vi "FPGA_Generate_PWM.vi"(10 "high-time (ticks)":i32, 11 "period(ticks)":i32) -> (3 "PWM out":bool)   [LabVIEW 2025]
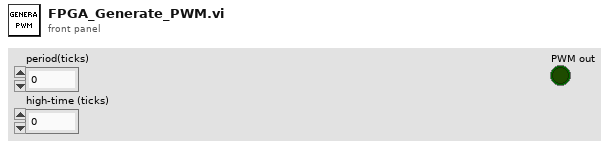
[diagram p1: front panel]
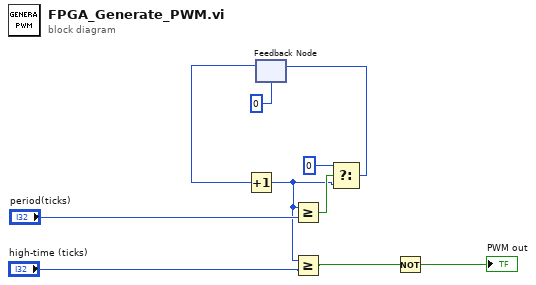
[diagram p0: block diagram]
diagram:
  n1 = feedback #1(0) -> (w9:i32)
  n2 = Increment(x=w9) -> (x+1=w4:i32)
  n3 = Greater Or Equal?(x=w4, y="period(ticks)") -> (x >= y?=w7:bool)
  n4 = Greater Or Equal?(x=w4, y="high-time (ticks)") -> (x >= y?=w2:bool)
  n5 = Select(t=0, s=w7, f=w4) -> (s? t:f=w5:i32)
  n6 = feedback-in #1(w5) -> ()
  n7 = Not(x=w2) -> (.not. x?=→"PWM out":bool)
